vi "Write Target Name.vi"(4 "Error In":errorcluster, 6 "Target Name":string, 7 "Remote Access Commands in":refnum<class "Remote Access Commands.lvclass">) -> (0 "Error Out":errorcluster, 3 "Remote Access Commands out":refnum<class "Remote Access Commands.lvclass">)   [LabVIEW 2015, in "Startup Processes.lvlib" / "Remote Access Commands.lvclass"]
uses:
  Remote Access Commands.lvclass
  Remote Access Commands.lvclass/Remote Access Commands.ctl
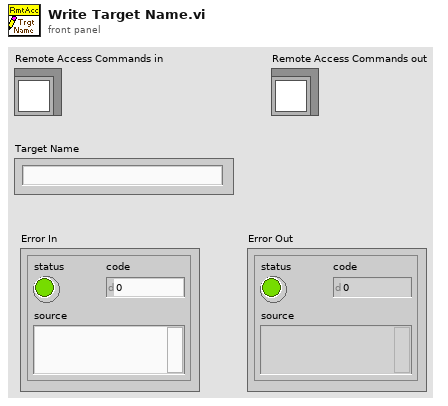
[diagram p1: front panel]
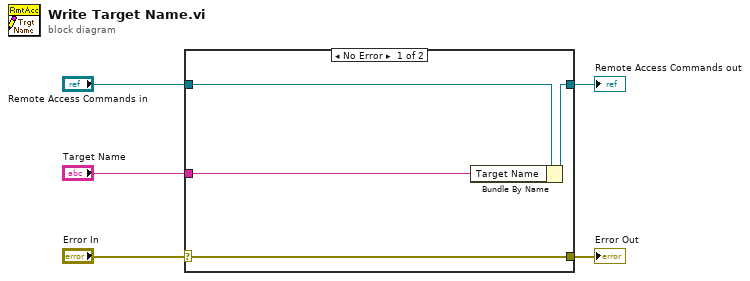
[diagram p0: block diagram]
diagram:
  n1 = case shown="No Error" "Error In" {
    selector: "Error In" -> [w9 w10]
    tunnel: [w9 w10] -> w4
    tunnel: [w7 w11] -> w2
    tunnel: "Remote Access Commands in" -> [w8 w11]
    tunnel: "Target Name" -> [w6 _]
    frame No Error {
      n2 = Bundle By Name(cluster=w8, "Target Name"=w6) -> (w7:refnum<class "Remote Access Commands.lvclass">)
    }
    frame Error {
    }
  }
  "Error Out" <- w4
  "Remote Access Commands out" <- w2
